vi "Alias to Q.vi"(10 "Alias":string, 11 "Self Actor in":refnum<class "Self Actor.lvclass">) -> (0 "error out":errorcluster, 1 "Alias found?":bool, 2 "Nest Msg Q":refnum<data-value>)   [LabVIEW 2021, in "LVCAM.lvlib" / "Self Actor.lvclass"]
uses:
  Self Actor.lvclass
  Msg Strategy/Msg Strategy.lvclass
  Self Actor.lvclass/Self Actor.ctl
  LVCAM.lvlib
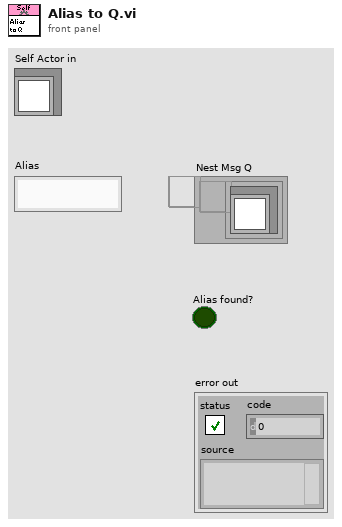
[diagram p1: front panel]
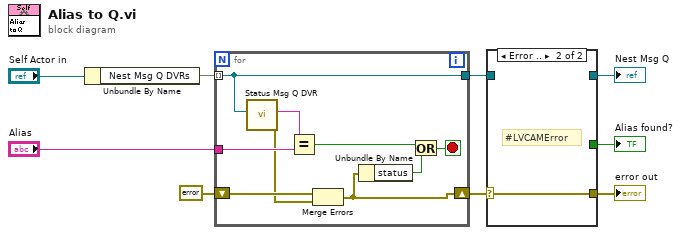
[diagram p0: block diagram]
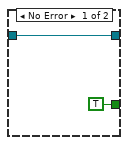
[diagram p2: hidden frame]
diagram:
  n1 = Unbundle By Name("Self Actor in") -> ("Nest Msg Q DVRs"=w8:set{refnum<data-value>})
  n2 = for {
    tunnel: w8 -> [w16] mode=indexing
    tunnel: [w16] -> w5
    tunnel: "Alias" -> [w17]
    shift-right: [w12] -> w4
    shift-left: errorcluster {"status"=FALSE, "code"=0, "source"=""} ("error out") -> [w18]
    stop <- w10 stop-if-true
    n3 = call "Status Msg Q DVR.vi"("Msg Q DVR"=w16) -> ("error out"=w14:errorcluster, "Msg Q DVR Alias"=w15:string)  [unwired: 9 in]
    n4 = Equal?(x=w15, y=w17) -> (x = y?=w13:bool)
    n5 = Merge Errors(w18, w14) -> (w12:errorcluster)
    n6 = Unbundle By Name(w12) -> ("status"=w11:bool)
    n7 = Or(x=w13, y=w11) -> (x .or. y?=w10:bool)
  }
  n8 = case shown="Error .." w4 {
    selector: w4 -> [_ w21]
    tunnel: w5 -> [w19 _]
    tunnel: [_ w21] -> w3
    tunnel: [TRUE ("Alias found?") _] -> w2
    tunnel: [w19 _] -> w1
    frame No Error {
    }
    frame Error {
      # "#LVCAMError"
    }
  }
  "error out" <- w3
  "Alias found?" <- w2
  "Nest Msg Q" <- w1
